vi "logEtaNData.vi"(0 "eta_iPath":path, 1 "time":dbl, 2 "eta":dbl[](array[numeric]), 3 "U":dbl[](array[numeric])) -> ()   [LabVIEW 2014]
uses:
  <vilib>/Utility/file.llb/Write To Spreadsheet File (DBL).vi
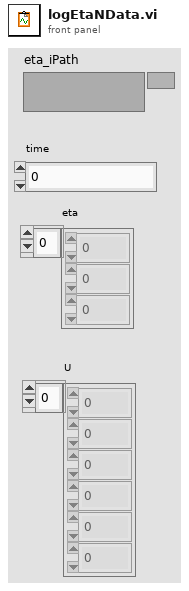
[diagram p1: front panel]
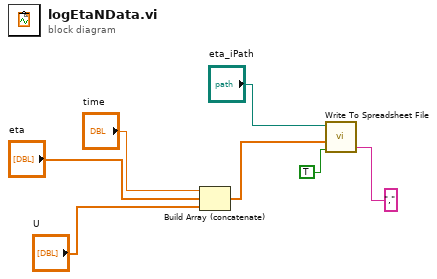
[diagram p0: block diagram]
diagram:
  n1 = Build Array (concatenate)("time", "eta", "U") -> (w5:dbl[])
  n2 = call-poly <vilib>:"Write To Spreadsheet File.vi"("delimiter (\\t)"="," ("delimiter (\\t)"), "append to file? (new file:F)"=TRUE, "1D data"=w5, "file path (dialog if empty)"="eta_iPath") -> ()  [unwired: 4 in, 1 out]
